vi "Get Control Properties.vi"(8 "error in":errorcluster, 11 "refnums in":refnum<vi>[](array[refnum])) -> (0 "error out":errorcluster, 1 "control indices":i32[](array[numeric]), 2 "labels":string[](array[string]), 3 "refnums out":refnum<vi>[](array[refnum]), 4 "class ids":u32[](array[numeric]), 6 "class names":string[](array[string]))   [LabVIEW 2020]
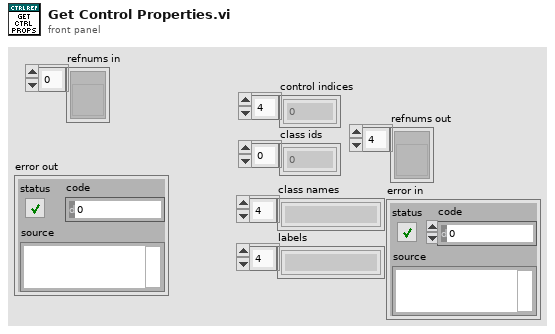
[diagram p1: front panel]
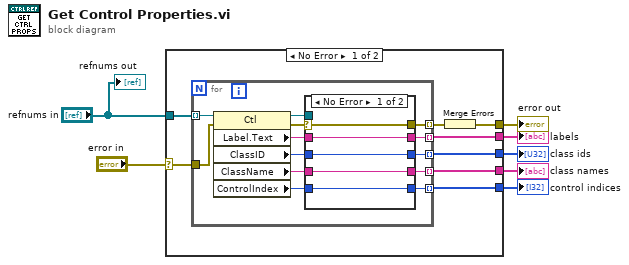
[diagram p0: block diagram]
diagram:
  n1 = case shown="No Error" "error in" {
    selector: "error in" -> [w8 w35]
    tunnel: "refnums in" -> [w14 _]
    tunnel: [w13 _] -> w6
    tunnel: [w12 _] -> w5
    tunnel: [w11 _] -> w4
    tunnel: [w10 _] -> w3
    tunnel: [w9 w35] -> w2
    frame No Error {
      n2 = for {
        tunnel: w14 -> [w28] mode=indexing
        tunnel: [w25] -> w10 mode=indexing
        tunnel: [w24] -> w11 mode=indexing
        tunnel: [w23] -> w12 mode=indexing
        tunnel: [w22] -> w13 mode=indexing
        tunnel: [w26] -> w15 mode=indexing
        tunnel: w8 -> [w16]
        n3 = property class="Ctl"(reference=w28, error in=w16) -> (reference out=w27:refnum<vi>, error out=w21:errorcluster, "Label.Text"=w20:string, "ClassID"=w19:u32, "ClassName"=w18:string, "ControlIndex"=w17:i32)
        n4 = case shown="No Error" w21 {
          selector: w21 -> [w33 w34]
          tunnel: w27 -> [_ _]
          tunnel: [w33 w34] -> w26
          tunnel: w20 -> [w32 _]
          tunnel: w19 -> [w31 _]
          tunnel: w18 -> [w30 _]
          tunnel: w17 -> [w29 _]
          tunnel: [w32 _] -> w25
          tunnel: [w31 _] -> w24
          tunnel: [w30 _] -> w23
          tunnel: [w29 _] -> w22
          frame No Error {
          }
          frame Error {
          }
        }
      }
      n5 = Merge Errors(w15) -> (w9:errorcluster)
    }
    frame Error {
    }
  }
  "error out" <- w2
  "control indices" <- w6
  "class names" <- w5
  "class ids" <- w4
  "labels" <- w3
  "refnums out" <- "refnums in"
